vi "SingleDeviceDServer.vi"() -> ()   [LabVIEW 2014, in "examples.lvlib"]
uses:
  examples.lvlib
  vis/tango_vi.llb/_TangoState_t.ctl
  vis/tango_vi.llb/_DServerClientRequest.ctl
  vis/tango_vi.llb/_DServerClientRequestType.ctl
  vis/tango_vi.llb/_DServerClientRequestData.ctl
  vis/tango_vi.llb/_GenericDataBuffer.ctl
  vis/tango_vi.llb/_AttributeDataType_t.ctl
  vis/tango_vi.llb/_LoggingLevel.ctl
  vis/tango_vi.llb/_DServerDevicePropertyToDouble.vi
  vis/tango_vi.llb/_DServerRequestDataToDevBoolean.vi
  vis/tango_vi.llb/_DServerRequestDataFromDevBoolean.vi
  vis/tango_vi.llb/_DServerRequestDataToDevCharArray.vi
  vis/tango_vi.llb/_DServerRequestDataFromDevCharArray.vi
  vis/tango_vi.llb/_DServerRequestDataToDevDouble.vi
  vis/tango_vi.llb/_DServerRequestDataFromDevDouble.vi
  vis/tango_vi.llb/_DServerRequestDataToDevDoubleArray.vi
  vis/tango_vi.llb/_DServerRequestDataFromDevDoubleArray.vi
  vis/tango_vi.llb/_DServerRequestDataToDevDoubleStringArray.vi
  vis/tango_vi.llb/_DServerRequestDataFromDevDoubleStringArray.vi
  vis/tango_vi.llb/_DServerRequestDataToDevFloat.vi
  vis/tango_vi.llb/_DServerRequestDataFromDevFloat.vi
  vis/tango_vi.llb/_DServerRequestDataToDevFloatArray.vi
  vis/tango_vi.llb/_DServerRequestDataFromDevFloatArray.vi
  vis/tango_vi.llb/_DServerRequestDataToDevLong.vi
  vis/tango_vi.llb/_DServerRequestDataFromDevLong.vi
  vis/tango_vi.llb/_DServerRequestDataToDevLong64.vi
  vis/tango_vi.llb/_DServerRequestDataFromDevLong64.vi
  vis/tango_vi.llb/_DServerRequestDataToDevLong64Array.vi
  vis/tango_vi.llb/_DServerRequestDataFromDevLong64Array.vi
  vis/tango_vi.llb/_DServerRequestDataToDevLongArray.vi
  vis/tango_vi.llb/_DServerRequestDataFromDevLongArray.vi
  vis/tango_vi.llb/_DServerRequestDataToDevLongStringArray.vi
  vis/tango_vi.llb/_DServerRequestDataFromDevLongStringArray.vi
  vis/tango_vi.llb/_DServerRequestDataToDevShort.vi
  vis/tango_vi.llb/_DServerRequestDataFromDevShort.vi
  vis/tango_vi.llb/_DServerRequestDataToDevEnum.vi
  vis/tango_vi.llb/_DServerRequestDataFromDevEnum.vi
  vis/tango_vi.llb/_DServerRequestDataToDevShortArray.vi
  vis/tango_vi.llb/_DServerRequestDataFromDevShortArray.vi
  vis/tango_vi.llb/_DServerRequestDataToDevString.vi
  vis/tango_vi.llb/_DServerRequestDataFromDevString.vi
  vis/tango_vi.llb/_DServerRequestDataToDevStringArray.vi
  vis/tango_vi.llb/_DServerRequestDataFromDevStringArray.vi
  vis/tango_vi.llb/_DServerRequestDataToDevULong.vi
  vis/tango_vi.llb/_DServerRequestDataFromDevULong.vi
  vis/tango_vi.llb/_DServerRequestDataToDevULong64.vi
  vis/tango_vi.llb/_DServerRequestDataFromDevULong64.vi
  vis/tango_vi.llb/_DServerRequestDataToDevULong64Array.vi
  vis/tango_vi.llb/_DServerRequestDataFromDevULong64Array.vi
  vis/tango_vi.llb/_DServerRequestDataToDevULongArray.vi
  vis/tango_vi.llb/_DServerRequestDataFromDevULongArray.vi
  vis/tango_vi.llb/_DServerRequestDataToDevUShort.vi
  vis/tango_vi.llb/_DServerRequestDataFromDevUShort.vi
  AttributesDataStorage.vi
  Common/UtilsRandomInstances/_UtilsRandom2DBoolArray.vi
  vis/tango_vi.llb/_DServerSetBooleanImageAttributeValue.vi
  vis/tango_vi.llb/_DServerSetBooleanScalarAttributeValue.vi
  Common/UtilsRandomInstances/_UtilsRandomBoolArray.vi
  vis/tango_vi.llb/_DServerSetBooleanSpectrumAttributeValue.vi
  Common/UtilsRandomInstances/_UtilsRandom2DDBLArray.vi
  vis/tango_vi.llb/_DServerSetDoubleImageAttributeValue.vi
  vis/tango_vi.llb/_DServerSetDoubleScalarAttributeValue.vi
  Common/UtilsRandomInstances/_UtilsRandomDBLArray.vi
  vis/tango_vi.llb/_DServerSetDoubleSpectrumAttributeValue.vi
  Common/UtilsRandomInstances/_UtilsRandomI16Value.vi
  vis/tango_vi.llb/_DServerSetUShortScalarAttributeValue.vi
  Common/UtilsRandomInstances/_UtilsRandom2DSGLArray.vi
  vis/tango_vi.llb/_DServerSetFloatImageAttributeValue.vi
  Common/UtilsRandomInstances/_UtilsRandomSGLValue.vi
  vis/tango_vi.llb/_DServerSetFloatScalarAttributeValue.vi
  Common/UtilsRandomInstances/_UtilsRandomSGLArray.vi
  vis/tango_vi.llb/_DServerSetFloatSpectrumAttributeValue.vi
  Common/UtilsRandomInstances/_UtilsRandom2DI64Array.vi
  vis/tango_vi.llb/_DServerSetLong64ImageAttributeValue.vi
  Common/UtilsRandomInstances/_UtilsRandomI64Value.vi
  vis/tango_vi.llb/_DServerSetLong64ScalarAttributeValue.vi
  Common/UtilsRandomInstances/_UtilsRandomI64Array.vi
  vis/tango_vi.llb/_DServerSetLong64SpectrumAttributeValue.vi
  Common/UtilsRandomInstances/_UtilsRandom2DI32Array.vi
  vis/tango_vi.llb/_DServerSetLongImageAttributeValue.vi
  Common/UtilsRandomInstances/_UtilsRandomI32Value.vi
  vis/tango_vi.llb/_DServerSetLongScalarAttributeValue.vi
  Common/UtilsRandomInstances/_UtilsRandomU32Array.vi
  vis/tango_vi.llb/_DServerSetLongSpectrumAttributeValue.vi
  Common/UtilsRandomInstances/_UtilsRandom2DI16Array.vi
  vis/tango_vi.llb/_DServerSetShortImageAttributeValue.vi
  vis/tango_vi.llb/_DServerSetEnumScalarAttributeValue.vi
  Common/UtilsRandomInstances/_UtilsRandomI16Array.vi
  vis/tango_vi.llb/_DServerSetShortSpectrumAttributeValue.vi
  vis/tango_vi.llb/_DServerSetStateImageAttributeValue.vi
  vis/tango_vi.llb/_DServerSetStateScalarAttributeValue.vi
  vis/tango_vi.llb/_DServerSetStateSpectrumAttributeValue.vi
  vis/tango_vi.llb/_DServerSetStringImageAttributeValue.vi
  Common/UtilsRandomInstances/_UtilsRandomStringValue.vi
  vis/tango_vi.llb/_DServerSetStringScalarAttributeValue.vi
  vis/tango_vi.llb/_DServerSetStringSpectrumAttributeValue.vi
  Common/UtilsRandomInstances/_UtilsRandom2DU8Array.vi
  vis/tango_vi.llb/_DServerSetUCharImageAttributeValue.vi
  Common/UtilsRandomInstances/_UtilsRandomU8Value.vi
  vis/tango_vi.llb/_DServerSetUCharScalarAttributeValue.vi
  Common/UtilsRandomInstances/_UtilsRandomU8Array.vi
  vis/tango_vi.llb/_DServerSetUCharSpectrumAttributeValue.vi
  Common/UtilsRandomInstances/_UtilsRandom2DU64Array.vi
  vis/tango_vi.llb/_DServerSetULong64ImageAttributeValue.vi
  Common/UtilsRandomInstances/_UtilsRandomU64Value.vi
  vis/tango_vi.llb/_DServerSetULong64ScalarAttributeValue.vi
  Common/UtilsRandomInstances/_UtilsRandomU64Array.vi
  vis/tango_vi.llb/_DServerSetULong64SpectrumAttributeValue.vi
  Common/UtilsRandomInstances/_UtilsRandom2DU32Array.vi
  vis/tango_vi.llb/_DServerSetULongImageAttributeValue.vi
  Common/UtilsRandomInstances/_UtilsRandomU32Value.vi
  vis/tango_vi.llb/_DServerSetULongScalarAttributeValue.vi
  Common/UtilsRandomInstances/_UtilsRandomI32Array.vi
  vis/tango_vi.llb/_DServerSetULongSpectrumAttributeValue.vi
  Common/UtilsRandomInstances/_UtilsRandom2DU16Array.vi
  vis/tango_vi.llb/_DServerSetUShortImageAttributeValue.vi
  Common/UtilsRandomInstances/_UtilsRandomU16Value.vi
  Common/UtilsRandomInstances/_UtilsRandomU16Array.vi
  vis/tango_vi.llb/_DServerSetUShortSpectrumAttributeValue.vi
  vis/tango_vi.llb/_DServerRequestDataToBooleanImage.vi
  vis/tango_vi.llb/_DServerRequestDataToBooleanScalar.vi
  vis/tango_vi.llb/_DServerRequestDataToBooleanSpectrum.vi
  vis/tango_vi.llb/_DServerRequestDataToDoubleImage.vi
  vis/tango_vi.llb/_DServerRequestDataToDoubleScalar.vi
  vis/tango_vi.llb/_DServerRequestDataToDoubleSpectrum.vi
  vis/tango_vi.llb/_DServerRequestDataToFloatImage.vi
  vis/tango_vi.llb/_DServerRequestDataToFloatScalar.vi
  vis/tango_vi.llb/_DServerRequestDataToFloatSpectrum.vi
  vis/tango_vi.llb/_DServerRequestDataToLong64Image.vi
  vis/tango_vi.llb/_DServerRequestDataToLong64Scalar.vi
  vis/tango_vi.llb/_DServerRequestDataToLong64Spectrum.vi
  vis/tango_vi.llb/_DServerRequestDataToLongImage.vi
  vis/tango_vi.llb/_DServerRequestDataToLongScalar.vi
  vis/tango_vi.llb/_DServerRequestDataToLongSpectrum.vi
  vis/tango_vi.llb/_DServerRequestDataToShortImage.vi
  vis/tango_vi.llb/_DServerRequestDataToShortScalar.vi
  vis/tango_vi.llb/_DServerRequestDataToEnumScalar.vi
  vis/tango_vi.llb/_DServerRequestDataToShortSpectrum.vi
  vis/tango_vi.llb/_DServerRequestDataToStateImage.vi
  vis/tango_vi.llb/_DServerRequestDataToStateScalar.vi
  vis/tango_vi.llb/_DServerRequestDataToStateSpectrum.vi
  vis/tango_vi.llb/_DServerRequestDataToStringImage.vi
  vis/tango_vi.llb/_DServerRequestDataToStringScalar.vi
  vis/tango_vi.llb/_DServerRequestDataToStringSpectrum.vi
  vis/tango_vi.llb/_DServerRequestDataToUCharImage.vi
  vis/tango_vi.llb/_DServerRequestDataToUCharScalar.vi
  vis/tango_vi.llb/_DServerRequestDataToUCharSpectrum.vi
  vis/tango_vi.llb/_DServerRequestDataToULong64Spectrum.vi
  vis/tango_vi.llb/_DServerRequestDataToULong64Scalar.vi
  vis/tango_vi.llb/_DServerRequestDataToULongImage.vi
  vis/tango_vi.llb/_DServerRequestDataToULongScalar.vi
  vis/tango_vi.llb/_DServerRequestDataToULongSpectrum.vi
  vis/tango_vi.llb/_DServerRequestDataToUShortImage.vi
  vis/tango_vi.llb/_DServerRequestDataToUShortScalar.vi
  vis/tango_vi.llb/_DServerRequestDataToUShortSpectrum.vi
  vis/tango_vi.llb/tango.lvlib
panel:
  in  "Device Tmo (in sec)":dbl=3.0
  out "Scale [Property Val.]":dbl
  out "Client Request":T1={"Request Id"=0, "Source Id"=0, "Request Type"=enum."UNKNOWN_REQUEST", "Device Class Name"="unspecified_class_name", "Device Name"="unspecified/device/name", "Cmd or Attr Name"="unspecified_cmd_or_attr_name", "Client Request Data"={"write attribute value"={"dimx"=0, "dimy"=0, "data"=[], "data_type"=enum."UNKNOWN_DATA_TYPE"}, "exec. command argin"={"num data"=[], "str data"=[]}}}
  out "State":T6=enum."UNKNOWN"
  out "Devive List":string[](array[string])
  in  "Instance Name":string="1"
  in  "Executable Name":string="LabviewSingleDeviceDServer"
  in  "devDoubleScalar":dbl(knob)=50.0 max=400.0 scale=0.0..100.0
  in  "?":bool
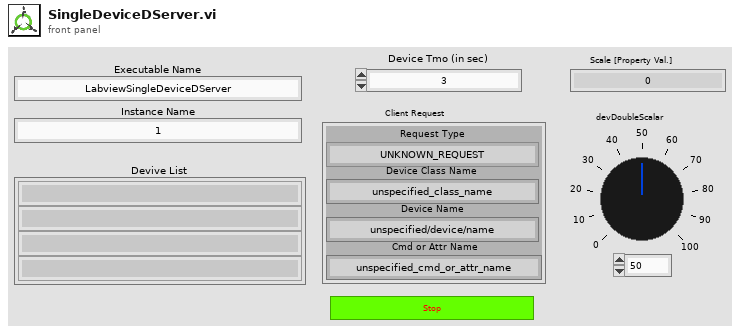
[diagram p1: front panel]
types:
  T1 = typedef "tango.lvlib/_DServerClientRequest.ctl" = cluster{"Request Id":u32, "Source Id":u32, "Request Type":T2, "Device Class Name":string, "Device Name":string, "Cmd or Attr Name":string, "Client Request Data":T3}
  T2 = typedef "tango.lvlib/_DServerClientRequestType.ctl" = enum16{"EXEC_CMD", "READ_ATTR", "WRITE_ATTR", "UNKNOWN_REQUEST"}
  T3 = typedef "tango.lvlib/_DServerClientRequestData.ctl" = cluster{"write attribute value":T4, "exec. command argin":cluster{"num data":u8[], "str data":string[]}}
  T4 = typedef "tango.lvlib/_GenericDataBuffer.ctl" = cluster{"dimx":u32, "dimy":u32, "data":u8[], "data_type":T5}
  T5 = typedef "tango.lvlib/_AttributeDataType_t.ctl" = enum16{"STATE_SCA", "STATE_SPE", "STATE_IMG", "STRING_SCA", "STRING_SPE", "STRING_IMG", "BOOL_SCA", "BOOL_SPE", "BOOL_IMG", "UCHAR_SCA", "UCHAR_SPE", "UCHAR_IMG", "SHORT_SCA", "SHORT_SPE", "SHORT_IMG", "USHORT_SCA", "USHORT_SPE", "USHORT_IMG", "LONG_SCA", "LONG_SPE", "LONG_IMG", "ULONG_SCA", "ULONG_SPE", "ULONG_IMG", "LONG64_SCA", "LONG64_SPE", "LONG64_IMG", "ULONG64_SCA", "ULONG64_SPE", "ULONG64_IMG", "FLOAT_SCA", "FLOAT_SPE", "FLOAT_IMG", "DOUBLE_SCA", "DOUBLE_SPE", "DOUBLE_IMG", "ENUM_SCA", "UNKNOWN_DATA_TYPE"}
  T6 = typedef "tango.lvlib/_TangoState_t.ctl" = enum32{"ON", "OFF", "CLOSE", "OPEN", "INSERT", "EXTRACT", "MOVING", "STANDBY", "FAULT", "INIT", "RUNNING", "ALARM", "DISABLE", "UNKNOWN"}
  T7 = typedef "tango.lvlib/_DServerEvent.ctl" = cluster{"event registration refnum":refnum<event-registration>, "user event out":refnum<user-event>}
  T8 = typedef "tango.lvlib/_LoggingLevel.ctl" = enum16{"DEBUG", "INFO", "WARNING", "ERROR", "FATAL"}
  T9 = enum16{"ENUM0", "ENUM1", "ENUM2", "ENUM3", "UNKNOWN"}
  T10 = cluster{"device name":string, "attribute name":string, "r/w access":i16, "format":i16, "data type":i16, "level":i16, "label":string, "unit":string, "display format":string, "min value":string, "max value":string, "min alarm":string, "max alarm":string}
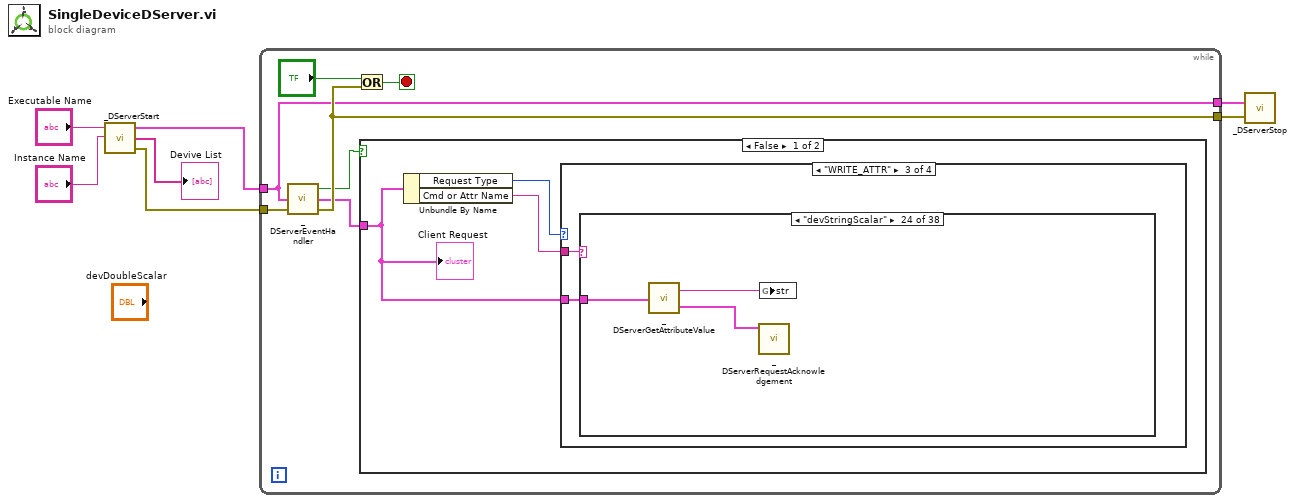
[diagram p0: block diagram]
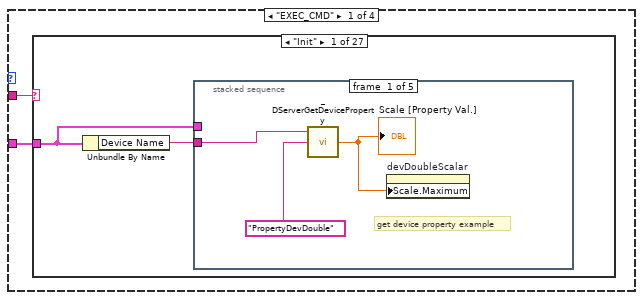
[diagram p2: hidden frame]
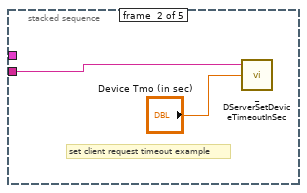
[diagram p3: hidden frame]
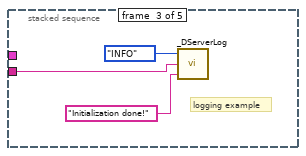
[diagram p4: hidden frame]
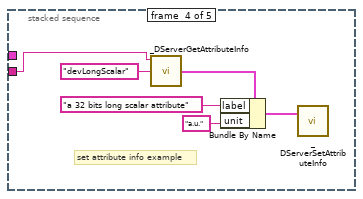
[diagram p5: hidden frame]
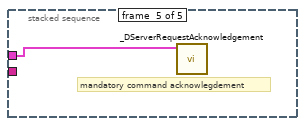
[diagram p6: hidden frame]
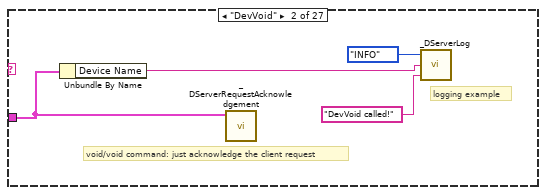
[diagram p7: hidden frame]
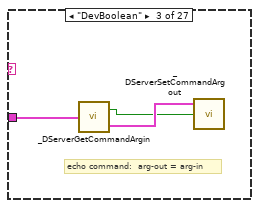
[diagram p8: hidden frame]
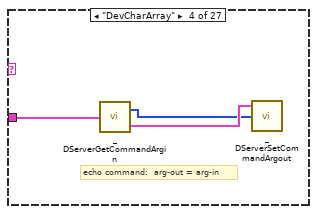
[diagram p9: hidden frame]
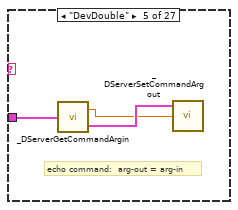
[diagram p10: hidden frame]
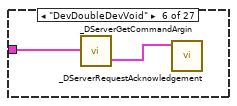
[diagram p11: hidden frame]
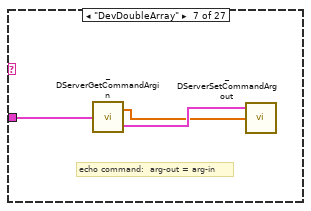
[diagram p12: hidden frame]
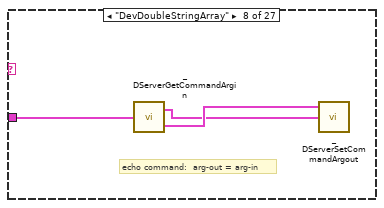
[diagram p13: hidden frame]
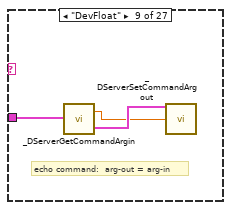
[diagram p14: hidden frame]
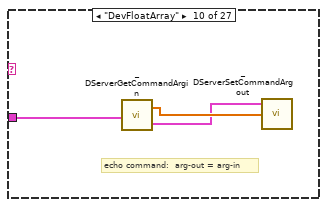
[diagram p15: hidden frame]
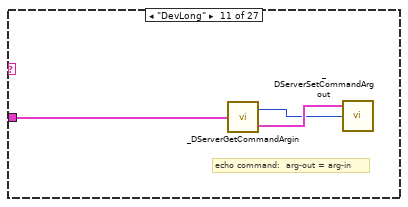
[diagram p16: hidden frame]
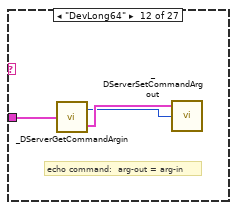
[diagram p17: hidden frame]
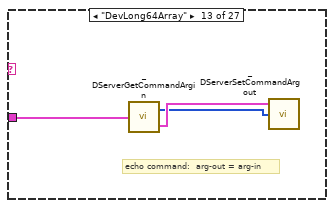
[diagram p18: hidden frame]
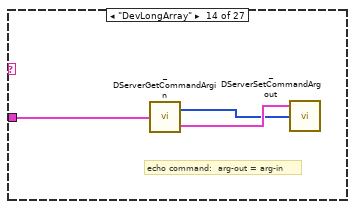
[diagram p19: hidden frame]
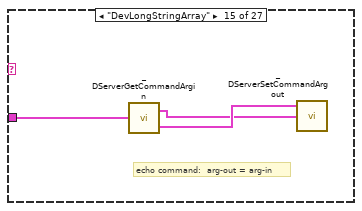
[diagram p20: hidden frame]
diagram:
  n1 = call "_DServerStart.vi"("instance name"="Instance Name", "executable name"="Executable Name") -> ("error out"=w5:errorcluster, "device_list"=→"Devive List":string[], "dserver evt."=w7:T7)  [unwired: 1 in]
  n2 = while {
    tunnel: w5 -> [w12]
    tunnel: w7 -> [w10]
    tunnel: [w11] -> w2
    tunnel: [w10] -> w1
    stop <- w14 stop-if-true
    n3 = call "_DServerEventHandler.vi"("error in"=w12, "dserver evt."=w10) -> ("error out"=w11:errorcluster, "client request"=w8:T1, "timeout"=w9:bool)  [unwired: 1 in]
    n4 = Or(x="?", y=w11) -> (x .or. y?=w14:bool)
    n5 = case shown="False" w9 {
      tunnel: w8 -> [w15 _]
      frame False {
        n6 = Unbundle By Name(w15) -> ("Request Type"=w16:T2, "Cmd or Attr Name"=w17:string)
        n7 = case shown="\"WRITE_ATTR\"" w16 {
          tunnel: w17 -> [w19 w114 w400 _]
          tunnel: w15 -> [w18 w113 w399 w513]
          frame "EXEC_CMD" {
            n8 = case shown="\"Init\"" w19 {
              tunnel: w18 -> [w20 w37 w41 w46 w49 w51 w54 w57 w60 w63 w64 w67 w71 w75 w76 w81 w84 w87 w90 w93 w96 w97 w102 w105 w108 w111 w112]
              frame "Init" {
                n9 = Unbundle By Name(w20) -> ("Device Name"=w21:string)
                n10 = stacked-sequence {
                  tunnel: w21 -> [w23 w25 w28 w32 _]
                  tunnel: w20 -> [_ _ _ _ w36]
                  frame #0 {
                    # "get device property example"
                    n11 = call-poly "_DServerGetDeviceProperty.vi"("property name"="PropertyDevDouble", "device name"=w23) -> ("property value"=w22:dbl)  [unwired: 2 in, 1 out]
                    "Scale [Property Val.]" <- w22
                    n12 = property on="devDoubleScalar" class="Knob (strict)"("Scale.Maximum"=w22) -> ()  [unwired: 2 in, 2 out]
                  }
                  frame #1 {
                    # "set client request timeout example"
                    n13 = call "_DServerSetDeviceTimeoutInSec.vi"("client request timeout in sec"="Device Tmo (in sec)", "device name"=w25) -> ()  [unwired: 3 in, 1 out]
                  }
                  frame #2 {
                    # "logging example"
                    n14 = call "_DServerLog.vi"("text"="Initialization done!", "device name"=w28, "logging level"=_LoggingLevel."INFO") -> ()  [unwired: 3 in]
                  }
                  frame #3 {
                    # "set attribute info example"
                    n15 = call "_DServerGetAttributeInfo.vi"("attribute name"="devLongScalar", "device name"=w32) -> ("attribute info"=w34:T10)  [unwired: 2 in, 1 out]
                    n16 = Bundle By Name(cluster=w34, "label"="a 32 bits long scalar attribute", "unit"="a.u.") -> (w33:T10)
                    n17 = call "_DServerSetAttributeInfo.vi"("attribute info"=w33) -> ()  [unwired: 2 in, 1 out]
                  }
                  frame #4 {
                    # "mandatory command acknowlegdement"
                    n18 = call "_DServerRequestAcknowledgement.vi"("client request"=w36) -> ()  [unwired: 6 in, 1 out]
                  }
                }
              }
              frame "DevVoid" {
                # "logging example"
                # "void/void command: just acknowledge the client request"
                n19 = Unbundle By Name(w37) -> ("Device Name"=w38:string)
                n20 = call "_DServerRequestAcknowledgement.vi"("client request"=w37) -> ()  [unwired: 6 in, 1 out]
                n21 = call "_DServerLog.vi"("text"="DevVoid called!", "device name"=w38, "logging level"=_LoggingLevel."INFO") -> ()  [unwired: 3 in]
              }
              frame "DevBoolean" {
                # "echo command:  arg-out = arg-in"
                n22 = call-poly "_DServerGetCommandArgin.vi"("client request"=w41) -> ("argin"=w42:bool, "client request"=w43:T1)
                n23 = call-poly "_DServerSetCommandArgout.vi"("argout value"=w42, "client request"=w43) -> ()  [unwired: 3 in, 1 out]
              }
              frame "DevCharArray" {
                # "echo command:  arg-out = arg-in"
                n24 = call-poly "_DServerGetCommandArgin.vi"("client request"=w46) -> ("argin"=w44:i8[], "client request"=w45:T1)
                n25 = call-poly "_DServerSetCommandArgout.vi"("argout value"=w44, "client request"=w45) -> ()  [unwired: 3 in, 1 out]
              }
              frame "DevDouble" {
                # "echo command:  arg-out = arg-in"
                n26 = call-poly "_DServerGetCommandArgin.vi"("client request"=w49) -> ("argin"=w47:dbl, "client request"=w48:T1)
                n27 = call-poly "_DServerSetCommandArgout.vi"("argout value"=w47, "client request"=w48) -> ()  [unwired: 3 in, 1 out]
              }
              frame "DevDoubleDevVoid" {
                n28 = call-poly "_DServerGetCommandArgin.vi"("client request"=w51) -> ("client request"=w50:T1)  [unwired: 1 out]
                n29 = call "_DServerRequestAcknowledgement.vi"("client request"=w50) -> ()  [unwired: 6 in, 1 out]
              }
              frame "DevDoubleArray" {
                # "echo command:  arg-out = arg-in"
                n30 = call-poly "_DServerGetCommandArgin.vi"("client request"=w54) -> ("argin"=w52:dbl[], "client request"=w53:T1)
                n31 = call-poly "_DServerSetCommandArgout.vi"("argout value"=w52, "client request"=w53) -> ()  [unwired: 3 in, 1 out]
              }
              frame "DevDoubleStringArray" {
                # "echo command:  arg-out = arg-in"
                n32 = call-poly "_DServerGetCommandArgin.vi"("client request"=w57) -> ("argin"=w55:cluster{"dvalue":dbl[], "svalue":string[]}, "client request"=w56:T1)
                n33 = call-poly "_DServerSetCommandArgout.vi"("argout value"=w55, "client request"=w56) -> ()  [unwired: 3 in, 1 out]
              }
              frame "DevFloat" {
                # "echo command:  arg-out = arg-in"
                n34 = call-poly "_DServerGetCommandArgin.vi"("client request"=w60) -> ("argin"=w58:sgl, "client request"=w59:T1)
                n35 = call-poly "_DServerSetCommandArgout.vi"("argout value"=w58, "client request"=w59) -> ()  [unwired: 3 in, 1 out]
              }
              frame "DevFloatArray" {
                # "echo command:  arg-out = arg-in"
                n36 = call-poly "_DServerGetCommandArgin.vi"("client request"=w63) -> ("argin"=w62:sgl[], "client request"=w61:T1)
                n37 = call-poly "_DServerSetCommandArgout.vi"("argout value"=w62, "client request"=w61) -> ()  [unwired: 3 in, 1 out]
              }
              frame "DevLong" {
                # "echo command:  arg-out = arg-in"
                n38 = call-poly "_DServerGetCommandArgin.vi"("client request"=w64) -> ("argin"=w65:i32, "client request"=w66:T1)
                n39 = call-poly "_DServerSetCommandArgout.vi"("argout value"=w65, "client request"=w66) -> ()  [unwired: 3 in, 1 out]
              }
              frame "DevLong64" {
                # "echo command:  arg-out = arg-in"
                n40 = call-poly "_DServerGetCommandArgin.vi"("client request"=w67) -> ("argin"=w68:i64, "client request"=w69:T1)
                n41 = call-poly "_DServerSetCommandArgout.vi"("argout value"=w68, "client request"=w69) -> ()  [unwired: 3 in, 1 out]
              }
              frame "DevLong64Array" {
                # "echo command:  arg-out = arg-in"
                n42 = call-poly "_DServerGetCommandArgin.vi"("client request"=w71) -> ("argin"=w70:i64[], "client request"=w72:T1)
                n43 = call-poly "_DServerSetCommandArgout.vi"("argout value"=w70, "client request"=w72) -> ()  [unwired: 3 in, 1 out]
              }
              frame "DevLongArray" {
                # "echo command:  arg-out = arg-in"
                n44 = call-poly "_DServerGetCommandArgin.vi"("client request"=w75) -> ("argin"=w73:i32[], "client request"=w74:T1)
                n45 = call-poly "_DServerSetCommandArgout.vi"("argout value"=w73, "client request"=w74) -> ()  [unwired: 3 in, 1 out]
              }
              frame "DevLongStringArray" {
                # "echo command:  arg-out = arg-in"
                n46 = call-poly "_DServerGetCommandArgin.vi"("client request"=w76) -> ("argin"=w77:cluster{"lvalue":i32[], "svalue":string[]}, "client request"=w78:T1)
                n47 = call-poly "_DServerSetCommandArgout.vi"("argout value"=w77, "client request"=w78) -> ()  [unwired: 3 in, 1 out]
              }
              frame "DevShort" {
                # "echo command:  arg-out = arg-in"
                n48 = call-poly "_DServerGetCommandArgin.vi"("client request"=w81) -> ("argin"=w79:i16, "client request"=w80:T1)
                n49 = call-poly "_DServerSetCommandArgout.vi"("argout value"=w79, "client request"=w80) -> ()  [unwired: 3 in, 1 out]
              }
              frame "DevEnum" {
                # "echo command:  arg-out = arg-in"
                n50 = call-poly "_DServerGetCommandArgin.vi"("client request"=w84) -> ("argin"=w82:i16, "client request"=w83:T1)
                n51 = call-poly "_DServerSetCommandArgout.vi"("argout value"=w82, "client request"=w83) -> ()  [unwired: 3 in, 1 out]
              }
              frame "DevShortArray" {
                # "echo command:  arg-out = arg-in"
                n52 = call-poly "_DServerGetCommandArgin.vi"("client request"=w87) -> ("argin"=w85:i16[], "client request"=w86:T1)
                n53 = call-poly "_DServerSetCommandArgout.vi"("argout value"=w85, "client request"=w86) -> ()  [unwired: 3 in, 1 out]
              }
              frame "DevString" {
                # "echo command:  arg-out = arg-in"
                n54 = call-poly "_DServerGetCommandArgin.vi"("client request"=w90) -> ("argin"=w88:string, "client request"=w89:T1)
                n55 = call-poly "_DServerSetCommandArgout.vi"("argout value"=w88, "client request"=w89) -> ()  [unwired: 3 in, 1 out]
              }
              frame "DevStringArray" {
                # "echo command:  arg-out = arg-in"
                n56 = call-poly "_DServerGetCommandArgin.vi"("client request"=w93) -> ("argin"=w91:string[], "client request"=w92:T1)
                n57 = call-poly "_DServerSetCommandArgout.vi"("argout value"=w91, "client request"=w92) -> ()  [unwired: 3 in, 1 out]
              }
              frame "DevULong" {
                # "echo command:  arg-out = arg-in"
                n58 = call-poly "_DServerGetCommandArgin.vi"("client request"=w96) -> ("argin"=w94:u32, "client request"=w95:T1)
                n59 = call-poly "_DServerSetCommandArgout.vi"("argout value"=w94, "client request"=w95) -> ()  [unwired: 3 in, 1 out]
              }
              frame "DevULong64" {
                # "echo command:  arg-out = arg-in"
                n60 = call-poly "_DServerGetCommandArgin.vi"("client request"=w97) -> ("argin"=w98:u64, "client request"=w99:T1)
                n61 = call-poly "_DServerSetCommandArgout.vi"("argout value"=w98, "client request"=w99) -> ()  [unwired: 3 in, 1 out]
              }
              frame "DevULong64Array" {
                # "echo command:  arg-out = arg-in"
                n62 = call-poly "_DServerGetCommandArgin.vi"("client request"=w102) -> ("argin"=w100:u64[], "client request"=w101:T1)
                n63 = call-poly "_DServerSetCommandArgout.vi"("argout value"=w100, "client request"=w101) -> ()  [unwired: 3 in, 1 out]
              }
              frame "DevULongArray" {
                # "echo command:  arg-out = arg-in"
                n64 = call-poly "_DServerGetCommandArgin.vi"("client request"=w105) -> ("argin"=w103:u32[], "client request"=w104:T1)
                n65 = call-poly "_DServerSetCommandArgout.vi"("argout value"=w103, "client request"=w104) -> ()  [unwired: 3 in, 1 out]
              }
              frame "DevUShort" {
                # "echo command:  arg-out = arg-in"
                n66 = call-poly "_DServerGetCommandArgin.vi"("client request"=w108) -> ("argin"=w106:u16, "client request"=w107:T1)
                n67 = call-poly "_DServerSetCommandArgout.vi"("argout value"=w106, "client request"=w107) -> ()  [unwired: 3 in, 1 out]
              }
              frame "DevUShortArray" {
                # "echo command:  arg-out = arg-in"
                n68 = call-poly "_DServerGetCommandArgin.vi"("client request"=w111) -> ("argin"=w109:i16[], "client request"=w110:T1)
                n69 = call-poly "_DServerSetCommandArgout.vi"("argout value"=w109, "client request"=w110) -> ()  [unwired: 3 in, 1 out]
              }
              frame Default {
                # "oops, this client request is not implemented"
                n70 = call "_DServerUnimplementedRequest.vi"("client request"=w112) -> ()  [unwired: 2 in, 1 out]
              }
            }
          }
          frame "READ_ATTR" {
            n71 = case shown="\"devBooleanImage\"" w114 {
              tunnel: w113 -> [w115 w124 w126 w133 w142 w144 w151 w160 w169 w175 w182 w191 w197 w204 w213 w219 w227 w235 w242 w248 w253 w255 w259 w271 w278 w288 w297 w304 w310 w319 w325 w332 w341 w347 w354 w363 w369 _ w376 w384 w392 w397 w398]
              frame "devBooleanImage" {
                # "return last written value or a random one in \n  case the attribute has never been written"
                n72 = global read "AttributesDataStorage.vi" "booli"() -> (w121:bool[][])
                n73 = Array Size(array=w121) -> (size(s)=w118:i32[])
                n74 = Index Array(array=w118, index=0) -> (element=w120:i32)
                n75 = Not Equal To 0?(x=w120) -> (x != 0?=w117:bool)
                n76 = case shown="False" w117 {
                  tunnel: [w122 w123] -> w116
                  tunnel: w121 -> [_ w123]
                  frame False {
                    n77 = call-poly "Random2DArray.vi"() -> ("random array"=w122:bool[][])  [unwired: 2 in]
                  }
                  frame True {
                  }
                }
                n78 = call-poly "_DServerSetAttributeValue.vi"("value"=w116, "client request"=w115) -> ()  [unwired: 3 in, 1 out]
              }
              frame "devBooleanScalar" {
                n79 = global read "AttributesDataStorage.vi" "bool"() -> (w125:bool)
                n80 = call-poly "_DServerSetAttributeValue.vi"(4:w125, "client request"=w124) -> ()  [unwired: 3 in, 1 out]
              }
              frame "devBooleanSpectrum" {
                # "return last written value or a random one in \n  case the attribute has never been written"
                n81 = global read "AttributesDataStorage.vi" "boolsp"() -> (w128:bool[])
                n82 = Array Size(array=w128) -> (size(s)=w129:i32)
                n83 = Not Equal To 0?(x=w129) -> (x != 0?=w130:bool)
                n84 = case shown="False" w130 {
                  tunnel: [w131 w132] -> w127
                  tunnel: w128 -> [_ w132]
                  frame False {
                    n85 = call-poly "Random1DArray.vi"() -> ("array"=w131:bool[])  [unwired: 2 in]
                  }
                  frame True {
                  }
                }
                n86 = call-poly "_DServerSetAttributeValue.vi"("value"=w127, "client request"=w126) -> ()  [unwired: 3 in, 1 out]
              }
              frame "devDoubleImage" {
                # "return last written value or a random one in \n  case the attribute has never been written"
                n87 = global read "AttributesDataStorage.vi" "dbli"() -> (w139:dbl[][])
                n88 = Array Size(array=w139) -> (size(s)=w136:i32[])
                n89 = Index Array(array=w136, index=0) -> (element=w138:i32)
                n90 = Not Equal To 0?(x=w138) -> (x != 0?=w135:bool)
                n91 = case shown="False" w135 {
                  tunnel: [w140 w141] -> w134
                  tunnel: w139 -> [_ w141]
                  frame False {
                    n92 = call-poly "Random2DArray.vi"() -> ("random array"=w140:dbl[][])  [unwired: 2 in]
                  }
                  frame True {
                  }
                }
                n93 = call-poly "_DServerSetAttributeValue.vi"("value"=w134, "client request"=w133) -> ()  [unwired: 3 in, 1 out]
              }
              frame "devDoubleScalar" {
                n94 = property on="devDoubleScalar" class="Knob (strict)"() -> ("Value"=w143:dbl)  [unwired: 2 in, 2 out]
                n95 = call-poly "_DServerSetAttributeValue.vi"("value"=w143, "client request"=w142) -> ()  [unwired: 3 in, 1 out]
              }
              frame "devDoubleSpectrum" {
                # "return last written value or a random one in \n  case the attribute has never been written"
                n96 = global read "AttributesDataStorage.vi" "dblsp"() -> (w146:dbl[])
                n97 = Array Size(array=w146) -> (size(s)=w147:i32)
                n98 = Not Equal To 0?(x=w147) -> (x != 0?=w148:bool)
                n99 = case shown="True" w148 {
                  tunnel: [w149 w150] -> w145
                  tunnel: w146 -> [_ w150]
                  frame False {
                    n100 = call-poly "Random1DArray.vi"() -> ("array"=w149:dbl[])  [unwired: 2 in]
                  }
                  frame True {
                  }
                }
                n101 = call-poly "_DServerSetAttributeValue.vi"("value"=w145, "client request"=w144) -> ()  [unwired: 3 in, 1 out]
              }
              frame "devEnumScalar" {
                # "return last written value or a random one in \n  case the attribute has never been written"
                n102 = global read "AttributesDataStorage.vi" "enum"() -> (w154:T9)
                n103 = Not Equal?(x=T9."UNKNOWN", y=w154) -> (x != y?=w155:bool)
                n104 = case shown="False" w155 {
                  tunnel: [w157 w159] -> w152
                  tunnel: w154 -> [_ w159]
                  frame False {
                    n105 = call-poly "RandomScalar.vi"() -> ("random value"=w158:i16)  [unwired: 1 in]
                    n106 = Quotient & Remainder(x=w158, y=T9."UNKNOWN" ("x")) -> (x-y*floor(x/y)=w157:u16)  [unwired: 1 out]
                  }
                  frame True {
                  }
                }
                n107 = call-poly "_DServerSetAttributeValue.vi"("value"=w152, "client request"=w151) -> ()  [unwired: 3 in, 1 out]
              }
              frame "devFloatImage" {
                # "return last written value or a random one in \n  case the attribute has never been written"
                n108 = global read "AttributesDataStorage.vi" "sgli"() -> (w166:sgl[][])
                n109 = Array Size(array=w166) -> (size(s)=w163:i32[])
                n110 = Index Array(array=w163, index=0) -> (element=w165:i32)
                n111 = Not Equal To 0?(x=w165) -> (x != 0?=w162:bool)
                n112 = case shown="False" w162 {
                  tunnel: [w167 w168] -> w161
                  tunnel: w166 -> [_ w168]
                  frame False {
                    n113 = call-poly "Random2DArray.vi"() -> ("random array"=w167:sgl[][])  [unwired: 2 in]
                  }
                  frame True {
                  }
                }
                n114 = call-poly "_DServerSetAttributeValue.vi"("value"=w161, "client request"=w160) -> ()  [unwired: 3 in, 1 out]
              }
              frame "devFloatScalar" {
                # "return last written value or a random one in \n  case the attribute has never been written"
                n115 = global read "AttributesDataStorage.vi" "sgl"() -> (w171:sgl)
                n116 = Not Equal To 0?(x=w171) -> (x != 0?=w172:bool)
                n117 = case shown="False" w172 {
                  tunnel: [w173 w174] -> w170
                  tunnel: w171 -> [_ w174]
                  frame False {
                    n118 = call-poly "RandomScalar.vi"() -> ("random value"=w173:sgl)  [unwired: 1 in]
                  }
                  frame True {
                  }
                }
                n119 = call-poly "_DServerSetAttributeValue.vi"("value"=w170, "client request"=w169) -> ()  [unwired: 3 in, 1 out]
              }
              frame "devFloatSpectrum" {
                # "return last written value or a random one in \n  case the attribute has never been written"
                n120 = global read "AttributesDataStorage.vi" "sglsp"() -> (w177:sgl[])
                n121 = Array Size(array=w177) -> (size(s)=w178:i32)
                n122 = Not Equal To 0?(x=w178) -> (x != 0?=w179:bool)
                n123 = case shown="False" w179 {
                  tunnel: [w180 w181] -> w176
                  tunnel: w177 -> [_ w181]
                  frame False {
                    n124 = call-poly "Random1DArray.vi"() -> ("array"=w180:sgl[])  [unwired: 2 in]
                  }
                  frame True {
                  }
                }
                n125 = call-poly "_DServerSetAttributeValue.vi"("value"=w176, "client request"=w175) -> ()  [unwired: 3 in, 1 out]
              }
              frame "devLong64Image" {
                # "return last written value or a random one in \n  case the attribute has never been written"
                n126 = global read "AttributesDataStorage.vi" "i64i"() -> (w188:i64[][])
                n127 = Array Size(array=w188) -> (size(s)=w185:i32[])
                n128 = Index Array(array=w185, index=0) -> (element=w187:i32)
                n129 = Not Equal To 0?(x=w187) -> (x != 0?=w184:bool)
                n130 = case shown="False" w184 {
                  tunnel: [w189 w190] -> w183
                  tunnel: w188 -> [_ w190]
                  frame False {
                    n131 = call-poly "Random2DArray.vi"() -> ("random array"=w189:i64[][])  [unwired: 2 in]
                  }
                  frame True {
                  }
                }
                n132 = call-poly "_DServerSetAttributeValue.vi"("value"=w183, "client request"=w182) -> ()  [unwired: 3 in, 1 out]
              }
              frame "devLong64Scalar" {
                # "return last written value or a random one in \n  case the attribute has never been written"
                n133 = global read "AttributesDataStorage.vi" "i64"() -> (w193:i64)
                n134 = Not Equal To 0?(x=w193) -> (x != 0?=w194:bool)
                n135 = case shown="False" w194 {
                  tunnel: [w195 w196] -> w192
                  tunnel: w193 -> [_ w196]
                  frame False {
                    n136 = call-poly "RandomScalar.vi"() -> ("random value"=w195:i64)  [unwired: 1 in]
                  }
                  frame True {
                  }
                }
                n137 = call-poly "_DServerSetAttributeValue.vi"("value"=w192, "client request"=w191) -> ()  [unwired: 3 in, 1 out]
              }
              frame "devLong64Spectrum" {
                # "return last written value or a random one in \n  case the attribute has never been written"
                n138 = global read "AttributesDataStorage.vi" "i64sp"() -> (w199:i64[])
                n139 = Array Size(array=w199) -> (size(s)=w200:i32)
                n140 = Not Equal To 0?(x=w200) -> (x != 0?=w201:bool)
                n141 = case shown="False" w201 {
                  tunnel: [w202 w203] -> w198
                  tunnel: w199 -> [_ w203]
                  frame False {
                    n142 = call-poly "Random1DArray.vi"() -> ("array"=w202:i64[])  [unwired: 2 in]
                  }
                  frame True {
                  }
                }
                n143 = call-poly "_DServerSetAttributeValue.vi"("value"=w198, "client request"=w197) -> ()  [unwired: 3 in, 1 out]
              }
              frame "devLongImage" {
                # "return last written value or a random one in \n  case the attribute has never been written"
                n144 = global read "AttributesDataStorage.vi" "i32i"() -> (w210:i32[][])
                n145 = Array Size(array=w210) -> (size(s)=w207:i32[])
                n146 = Index Array(array=w207, index=0) -> (element=w209:i32)
                n147 = Not Equal To 0?(x=w209) -> (x != 0?=w206:bool)
                n148 = case shown="False" w206 {
                  tunnel: [w211 w212] -> w205
                  tunnel: w210 -> [_ w212]
                  frame False {
                    n149 = call-poly "Random2DArray.vi"() -> ("random array"=w211:i32[][])  [unwired: 2 in]
                  }
                  frame True {
                  }
                }
                n150 = call-poly "_DServerSetAttributeValue.vi"("value"=w205, "client request"=w204) -> ()  [unwired: 3 in, 1 out]
              }
              frame "devLongScalar" {
                # "return last written value or a random one in \n  case the attribute has never been written"
                n151 = global read "AttributesDataStorage.vi" "i32"() -> (w214:i32)
                n152 = Not Equal To 0?(x=w214) -> (x != 0?=w216:bool)
                n153 = case shown="False" w216 {
                  tunnel: [w217 w218] -> w215
                  tunnel: w214 -> [_ w218]
                  frame False {
                    n154 = call-poly "RandomScalar.vi"() -> ("random value"=w217:i32)  [unwired: 1 in]
                  }
                  frame True {
                  }
                }
                n155 = call-poly "_DServerSetAttributeValue.vi"("value"=w215, "client request"=w213) -> ()  [unwired: 3 in, 1 out]
              }
              frame "devLongSpectrum" {
                # "return last written value or a random one in \n  case the attribute has never been written"
                n156 = global read "AttributesDataStorage.vi" "i32sp"() -> (w221:i32[])
                n157 = Array Size(array=w221) -> (size(s)=w222:i32)
                n158 = Not Equal To 0?(x=w222) -> (x != 0?=w223:bool)
                n159 = case shown="False" w223 {
                  tunnel: [w224 w225] -> w220
                  tunnel: w221 -> [_ w225]
                  frame False {
                    n160 = call-poly "Random1DArray.vi"() -> ("array"=w224:i32[])  [unwired: 2 in]
                  }
                  frame True {
                  }
                }
                n161 = call-poly "_DServerSetAttributeValue.vi"("value"=w220, "client request"=w219) -> ()  [unwired: 3 in, 1 out]
              }
              frame "devShortImage" {
                # "return last written value or a random one in \n  case the attribute has never been written"
                n162 = global read "AttributesDataStorage.vi" "i16i"() -> (w232:i16[][])
                n163 = Array Size(array=w232) -> (size(s)=w229:i32[])
                n164 = Index Array(array=w229, index=0) -> (element=w231:i32)
                n165 = Not Equal To 0?(x=w231) -> (x != 0?=w228:bool)
                n166 = case shown="False" w228 {
                  tunnel: [w233 w234] -> w226
                  tunnel: w232 -> [_ w234]
                  frame False {
                    n167 = call-poly "Random2DArray.vi"() -> ("random array"=w233:i16[][])  [unwired: 2 in]
                  }
                  frame True {
                  }
                }
                n168 = call-poly "_DServerSetAttributeValue.vi"("value"=w226, "client request"=w227) -> ()  [unwired: 3 in, 1 out]
              }
              frame "devShortScalar" {
                # "return last written value or a random one in \n  case the attribute has never been written"
                n169 = global read "AttributesDataStorage.vi" "i16"() -> (w237:i16)
                n170 = Not Equal To 0?(x=w237) -> (x != 0?=w238:bool)
                n171 = case shown="False" w238 {
                  tunnel: [w239 w240] -> w236
                  tunnel: w237 -> [_ w240]
                  frame False {
                    n172 = call-poly "RandomScalar.vi"() -> ("random value"=w239:i16)  [unwired: 1 in]
                  }
                  frame True {
                  }
                }
                n173 = call-poly "_DServerSetAttributeValue.vi"("value"=w236, "client request"=w235) -> ()  [unwired: 3 in, 1 out]
              }
              frame "devShortSpectrum" {
                # "return last written value or a random one in \n  case the attribute has never been written"
                n174 = global read "AttributesDataStorage.vi" "i16sp"() -> (w243:i16[])
                n175 = Array Size(array=w243) -> (size(s)=w244:i32)
                n176 = Not Equal To 0?(x=w244) -> (x != 0?=w245:bool)
                n177 = case shown="False" w245 {
                  tunnel: [w246 w247] -> w241
                  tunnel: w243 -> [_ w247]
                  frame False {
                    n178 = call-poly "Random1DArray.vi"() -> ("array"=w246:i16[])  [unwired: 2 in]
                  }
                  frame True {
                  }
                }
                n179 = call-poly "_DServerSetAttributeValue.vi"("value"=w241, "client request"=w242) -> ()  [unwired: 3 in, 1 out]
              }
              frame "devStateImage" {
                n180 = global read "AttributesDataStorage.vi" "state"() -> (w250:T6)
                n181 = Initialize Array(w250, 32 ("dimension size"), 32 ("dimension size")) -> (w249:T6[][])
                n182 = call-poly "_DServerSetAttributeValue.vi"("value"=w249, "client request"=w248) -> ()  [unwired: 3 in, 1 out]
              }
              frame "devStateScalar" {
                n183 = global read "AttributesDataStorage.vi" "state"() -> (w254:T6)
                n184 = call-poly "_DServerSetAttributeValue.vi"("value"=w254, "client request"=w253) -> ()  [unwired: 3 in, 1 out]
              }
              frame "devStateSpectrum" {
                n185 = global read "AttributesDataStorage.vi" "state"() -> (w257:T6)
                n186 = Initialize Array(w257, 32 ("dimension size")) -> (w256:T6[])
                n187 = call-poly "_DServerSetAttributeValue.vi"("value"=w256, "client request"=w255) -> ()  [unwired: 3 in, 1 out]
              }
              frame "devStringImage" {
                # "return last written value or a random one in \n  case the attribute has never been written"
                n188 = global read "AttributesDataStorage.vi" "stri"() -> (w265:string[][])
                n189 = Array Size(array=w265) -> (size(s)=w262:i32[])
                n190 = Index Array(array=w262, index=0) -> (element=w264:i32)
                n191 = Not Equal To 0?(x=w264) -> (x != 0?=w261:bool)
                n192 = case shown="False" w261 {
                  tunnel: [w266 w270] -> w260
                  tunnel: w265 -> [_ w270]
                  frame False {
                    w267 = 32 ("dimension size")
                    n193 = call "RandomValue.vi"() -> ("random value"=w269:dbl)  [unwired: 1 in]
                    n194 = Number To Hexadecimal String(2:w269) -> (0:w268:string)  [unwired: 1 in]
                    n195 = Initialize Array(w268, w267, w267) -> (w266:string[][])
                  }
                  frame True {
                  }
                }
                n196 = call-poly "_DServerSetAttributeValue.vi"("value"=w260, "client request"=w259) -> ()  [unwired: 3 in, 1 out]
              }
              frame "devStringScalar" {
                # "return last written value or a random one in \n  case the attribute has never been written"
                n197 = global read "AttributesDataStorage.vi" "str"() -> (w275:string)
                n198 = String Length(string=w275) -> (length=w273:i32)
                n199 = Not Equal To 0?(x=w273) -> (x != 0?=w274:bool)
                n200 = case shown="False" w274 {
                  tunnel: [w276 w277] -> w272
                  tunnel: w275 -> [_ w277]
                  frame False {
                    n201 = call-poly "RandomScalar.vi"() -> ("random value"=w276:string)  [unwired: 1 in]
                  }
                  frame True {
                  }
                }
                n202 = call-poly "_DServerSetAttributeValue.vi"("value"=w272, "client request"=w271) -> ()  [unwired: 3 in, 1 out]
              }
              frame "devStringSpectrum" {
                # "return last written value or a random one in \n  case the attribute has never been written"
                n203 = global read "AttributesDataStorage.vi" "strsp"() -> (w282:string[])
                n204 = Array Size(array=w282) -> (size(s)=w281:i32)
                n205 = Not Equal To 0?(x=w281) -> (x != 0?=w280:bool)
                n206 = case shown="True" w280 {
                  tunnel: [w283 w287] -> w279
                  tunnel: w282 -> [_ w287]
                  frame False {
                    n207 = call "RandomValue.vi"() -> ("random value"=w285:dbl)  [unwired: 1 in]
                    n208 = Number To Hexadecimal String(2:w285) -> (0:w284:string)  [unwired: 1 in]
                    n209 = Initialize Array(w284, 32 ("dimension size")) -> (w283:string[])
                  }
                  frame True {
                  }
                }
                n210 = call-poly "_DServerSetAttributeValue.vi"("value"=w279, "client request"=w278) -> ()  [unwired: 3 in, 1 out]
              }
              frame "devUCharImage" {
                # "return last written value or a random one in \n  case the attribute has never been written"
                n211 = global read "AttributesDataStorage.vi" "u8i"() -> (w294:u8[][])
                n212 = Array Size(array=w294) -> (size(s)=w291:i32[])
                n213 = Index Array(array=w291, index=0) -> (element=w293:i32)
                n214 = Not Equal To 0?(x=w293) -> (x != 0?=w290:bool)
                n215 = case shown="False" w290 {
                  tunnel: [w295 w296] -> w289
                  tunnel: w294 -> [_ w296]
                  frame False {
                    n216 = call-poly "Random2DArray.vi"() -> ("random array"=w295:u8[][])  [unwired: 2 in]
                  }
                  frame True {
                  }
                }
                n217 = call-poly "_DServerSetAttributeValue.vi"("value"=w289, "client request"=w288) -> ()  [unwired: 3 in, 1 out]
              }
              frame "devUCharScalar" {
                # "return last written value or a random one in \n  case the attribute has never been written"
                n218 = global read "AttributesDataStorage.vi" "u8"() -> (w298:u8)
                n219 = Not Equal To 0?(x=w298) -> (x != 0?=w300:bool)
                n220 = case shown="False" w300 {
                  tunnel: [w301 w302] -> w299
                  tunnel: w298 -> [_ w302]
                  frame False {
                    n221 = call-poly "RandomScalar.vi"() -> ("random value"=w301:u8)  [unwired: 1 in]
                  }
                  frame True {
                  }
                }
                n222 = call-poly "_DServerSetAttributeValue.vi"("value"=w299, "client request"=w297) -> ()  [unwired: 3 in, 1 out]
              }
              frame "devUCharSpectrum" {
                # "return last written value or a random one in \n  case the attribute has never been written"
                n223 = global read "AttributesDataStorage.vi" "u8sp"() -> (w305:u8[])
                n224 = Array Size(array=w305) -> (size(s)=w306:i32)
                n225 = Not Equal To 0?(x=w306) -> (x != 0?=w307:bool)
                n226 = case shown="False" w307 {
                  tunnel: [w308 w309] -> w303
                  tunnel: w305 -> [_ w309]
                  frame False {
                    n227 = call-poly "Random1DArray.vi"() -> ("array"=w308:u8[])  [unwired: 2 in]
                  }
                  frame True {
                  }
                }
                n228 = call-poly "_DServerSetAttributeValue.vi"("value"=w303, "client request"=w304) -> ()  [unwired: 3 in, 1 out]
              }
              frame "devULong64Image" {
                # "return last written value or a random one in \n  case the attribute has never been written"
                n229 = global read "AttributesDataStorage.vi" "u64i"() -> (w316:u64[][])
                n230 = Array Size(array=w316) -> (size(s)=w313:i32[])
                n231 = Index Array(array=w313, index=0) -> (element=w315:i32)
                n232 = Not Equal To 0?(x=w315) -> (x != 0?=w312:bool)
                n233 = case shown="False" w312 {
                  tunnel: [w317 w318] -> w311
                  tunnel: w316 -> [_ w318]
                  frame False {
                    n234 = call-poly "Random2DArray.vi"() -> ("random array"=w317:i64[][])  [unwired: 2 in]
                  }
                  frame True {
                  }
                }
                n235 = call-poly "_DServerSetAttributeValue.vi"("value"=w311, "client request"=w310) -> ()  [unwired: 3 in, 1 out]
              }
              frame "devULong64Scalar" {
                # "return last written value or a random one in \n  case the attribute has never been written"
                n236 = global read "AttributesDataStorage.vi" "u64"() -> (w321:u64)
                n237 = Not Equal To 0?(x=w321) -> (x != 0?=w322:bool)
                n238 = case shown="False" w322 {
                  tunnel: [w323 w324] -> w320
                  tunnel: w321 -> [_ w324]
                  frame False {
                    n239 = call-poly "RandomScalar.vi"() -> ("random value"=w323:u64)  [unwired: 1 in]
                  }
                  frame True {
                  }
                }
                n240 = call-poly "_DServerSetAttributeValue.vi"("value"=w320, "client request"=w319) -> ()  [unwired: 3 in, 1 out]
              }
              frame "devULong64Spectrum" {
                # "return last written value or a random one in \n  case the attribute has never been written"
                n241 = global read "AttributesDataStorage.vi" "u64sp"() -> (w327:u64[])
                n242 = Array Size(array=w327) -> (size(s)=w328:i32)
                n243 = Not Equal To 0?(x=w328) -> (x != 0?=w329:bool)
                n244 = case shown="False" w329 {
                  tunnel: [w330 w331] -> w326
                  tunnel: w327 -> [_ w331]
                  frame False {
                    n245 = call-poly "Random1DArray.vi"() -> ("array"=w330:u64[])  [unwired: 2 in]
                  }
                  frame True {
                  }
                }
                n246 = call-poly "_DServerSetAttributeValue.vi"("value"=w326, "client request"=w325) -> ()  [unwired: 3 in, 1 out]
              }
              frame "devULongImage" {
                # "return last written value or a random one in \n  case the attribute has never been written"
                n247 = global read "AttributesDataStorage.vi" "u32i"() -> (w338:u32[][])
                n248 = Array Size(array=w338) -> (size(s)=w335:i32[])
                n249 = Index Array(array=w335, index=0) -> (element=w337:i32)
                n250 = Not Equal To 0?(x=w337) -> (x != 0?=w334:bool)
                n251 = case shown="False" w334 {
                  tunnel: [w339 w340] -> w333
                  tunnel: w338 -> [_ w340]
                  frame False {
                    n252 = call-poly "Random2DArray.vi"() -> ("random array"=w339:u32[][])  [unwired: 2 in]
                  }
                  frame True {
                  }
                }
                n253 = call-poly "_DServerSetAttributeValue.vi"("value"=w333, "client request"=w332) -> ()  [unwired: 3 in, 1 out]
              }
              frame "devULongScalar" {
                # "return last written value or a random one in \n  case the attribute has never been written"
                n254 = global read "AttributesDataStorage.vi" "u32"() -> (w343:u32)
                n255 = Not Equal To 0?(x=w343) -> (x != 0?=w344:bool)
                n256 = case shown="False" w344 {
                  tunnel: [w345 w346] -> w342
                  tunnel: w343 -> [_ w346]
                  frame False {
                    n257 = call-poly "RandomScalar.vi"() -> ("random value"=w345:u32)  [unwired: 1 in]
                  }
                  frame True {
                  }
                }
                n258 = call-poly "_DServerSetAttributeValue.vi"("value"=w342, "client request"=w341) -> ()  [unwired: 3 in, 1 out]
              }
              frame "devULongSpectrum" {
                # "return last written value or a random one in \n  case the attribute has never been written"
                n259 = global read "AttributesDataStorage.vi" "u32sp"() -> (w349:u32[])
                n260 = Array Size(array=w349) -> (size(s)=w350:i32)
                n261 = Not Equal To 0?(x=w350) -> (x != 0?=w351:bool)
                n262 = case shown="False" w351 {
                  tunnel: [w352 w353] -> w348
                  tunnel: w349 -> [_ w353]
                  frame False {
                    n263 = call-poly "Random1DArray.vi"() -> ("array"=w352:u32[])  [unwired: 2 in]
                  }
                  frame True {
                  }
                }
                n264 = call-poly "_DServerSetAttributeValue.vi"("value"=w348, "client request"=w347) -> ()  [unwired: 3 in, 1 out]
              }
              frame "devUShortImage" {
                # "return last written value or a random one in \n  case the attribute has never been written"
                n265 = global read "AttributesDataStorage.vi" "u16i"() -> (w360:u16[][])
                n266 = Array Size(array=w360) -> (size(s)=w357:i32[])
                n267 = Index Array(array=w357, index=0) -> (element=w359:i32)
                n268 = Not Equal To 0?(x=w359) -> (x != 0?=w356:bool)
                n269 = case shown="False" w356 {
                  tunnel: [w361 w362] -> w355
                  tunnel: w360 -> [_ w362]
                  frame False {
                    n270 = call-poly "Random2DArray.vi"() -> ("random array"=w361:u16[][])  [unwired: 2 in]
                  }
                  frame True {
                  }
                }
                n271 = call-poly "_DServerSetAttributeValue.vi"("value"=w355, "client request"=w354) -> ()  [unwired: 3 in, 1 out]
              }
              frame "devUShortScalar" {
                # "return last written value or a random one in \n  case the attribute has never been written"
                n272 = global read "AttributesDataStorage.vi" "u16"() -> (w365:u16)
                n273 = Not Equal To 0?(x=w365) -> (x != 0?=w366:bool)
                n274 = case shown="False" w366 {
                  tunnel: [w367 w368] -> w364
                  tunnel: w365 -> [_ w368]
                  frame False {
                    n275 = call-poly "RandomScalar.vi"() -> ("random value"=w367:u16)  [unwired: 1 in]
                  }
                  frame True {
                  }
                }
                n276 = call-poly "_DServerSetAttributeValue.vi"("value"=w364, "client request"=w363) -> ()  [unwired: 3 in, 1 out]
              }
              frame "devUShortSpectrum" {
                # "return last written value or a random one in \n  case the attribute has never been written"
                n277 = global read "AttributesDataStorage.vi" "u16sp"() -> (w371:u16[])
                n278 = Array Size(array=w371) -> (size(s)=w372:i32)
                n279 = Not Equal To 0?(x=w372) -> (x != 0?=w373:bool)
                n280 = case shown="False" w373 {
                  tunnel: [w374 w375] -> w370
                  tunnel: w371 -> [_ w375]
                  frame False {
                    n281 = call-poly "Random1DArray.vi"() -> ("array"=w374:u16[])  [unwired: 2 in]
                  }
                  frame True {
                  }
                }
                n282 = call-poly "_DServerSetAttributeValue.vi"("value"=w370, "client request"=w369) -> ()  [unwired: 3 in, 1 out]
              }
              frame "noReplyAttribute" {
                # "we voluntarily don't reply to this request in order to observe the behavior of the Tango binding to such a situation - we expect the waiter (i.e. the thread handling the client request) to timeout and leave the place - the tango device will block (i.e. will not be able to handle another request) until the timeout expires - we consequently understand easily why we should reply to any single request - see _DServerRequestAcknowledgement.vi  -  the _DServerUnimplementedRequest.vi can also be temporary used to deal with \"not yet implemented\" features - see the \"default\" case for an example"
              }
              frame "slowReplyAttribute" {
                # "delay reply to see the timeout mechanism in action"
                n283 = flat-sequence {
                  tunnel: [w378] -> w377
                  tunnel: w376 -> [w378]
                  tunnel: w377 -> [w382]
                  frame #0 {
                    n284 = property on="Device Tmo (in sec)" class="DigNum (strict)"() -> ("Value"=w381:dbl)  [unwired: 2 in, 2 out]
                    n285 = Multiply(x=w381, y=1000.0) -> (x*y=w379:dbl)
                    n286 = Wait (ms)(milliseconds to wait=w379) -> ()  [unwired: 1 out]
                  }
                  frame #1 {
                    n287 = call-poly "Random1DArray.vi"() -> ("array"=w383:i32[])  [unwired: 2 in]
                    n288 = call-poly "_DServerSetAttributeValue.vi"("value"=w383, "client request"=w382) -> ()  [unwired: 3 in, 1 out]
                  }
                }
              }
              frame "State" {
                # "pseudo random state"
                n289 = Tick Count (ms)() -> (millisecond timer value=w386:u32)
                n290 = Quotient & Remainder(x=w386, y=u32 2) -> (x-y*floor(x/y)=w388:u32)  [unwired: 1 out]
                n291 = Equal To 0?(x=w388) -> (x = 0?=w387:bool)
                n292 = case shown="True" w387 {
                  tunnel: [_TangoState_t."OFF" ("Tango Device State") _TangoState_t."ON" ("Tango Device State")] -> w385
                  frame False {
                  }
                  frame True {
                  }
                }
                "State" <- w385
                n293 = call-poly "_DServerSetAttributeValue.vi"("value"=w385, "client request"=w384) -> ()  [unwired: 3 in, 1 out]
              }
              frame "Status" {
                n294 = property on="Tango Device State 1.1" class="Enum (strict)"() -> ("Value"=w394:T6)  [unwired: 2 in, 2 out]
                n295 = call "_TangoStateName.vi"("State"=w394) -> ("State Name"=w393:string)
                n296 = call-poly "_DServerSetAttributeValue.vi"("value"=w393, "client request"=w392) -> ()  [unwired: 3 in, 1 out]
              }
              frame "systematicErrorAttribute" {
                # "the acknowledgement VI can also be used to throw an \nexception that will be caught by the Tango client"
                n297 = call "_DServerRequestAcknowledgement.vi"("error string"="this is a systematic error!", "error code"=-1, "client request"=w397) -> ()  [unwired: 4 in, 1 out]
              }
              frame Default {
                # "oops, this client request is not implemented"
                n298 = call "_DServerUnimplementedRequest.vi"("client request"=w398) -> ()  [unwired: 2 in, 1 out]
              }
            }
          }
          frame "WRITE_ATTR" {
            n299 = case shown="\"devStringScalar\"" w400 {
              tunnel: w399 -> [w401 w404 w407 w410 w413 w416 w419 w422 w425 w428 w431 w434 w437 w440 w443 w446 w449 w452 w455 w458 w461 w464 w467 w471 w473 w476 w479 w482 w485 w488 w491 w494 w497 w500 w503 w506 w509 w512]
              frame "devBooleanImage" {
                n300 = call-poly "_DServerGetAttributeValue.vi"("client request"=w401) -> ("attribute value"=w403:bool[][], "client request"=w402:T1)
                n301 = call "_DServerRequestAcknowledgement.vi"("client request"=w402) -> ()  [unwired: 6 in, 1 out]
                n302 = global write "AttributesDataStorage.vi" "booli"(w403) -> ()
              }
              frame "devBooleanScalar" {
                n303 = call-poly "_DServerGetAttributeValue.vi"("client request"=w404) -> ("attribute value"=w406:bool, "client request"=w405:T1)
                n304 = call "_DServerRequestAcknowledgement.vi"("client request"=w405) -> ()  [unwired: 6 in, 1 out]
                n305 = global write "AttributesDataStorage.vi" "bool"(w406) -> ()
              }
              frame "devBooleanSpectrum" {
                n306 = call-poly "_DServerGetAttributeValue.vi"("client request"=w407) -> ("attribute value"=w409:bool[], "client request"=w408:T1)
                n307 = call "_DServerRequestAcknowledgement.vi"("client request"=w408) -> ()  [unwired: 6 in, 1 out]
                n308 = global write "AttributesDataStorage.vi" "boolsp"(w409) -> ()
              }
              frame "devDoubleImage" {
                n309 = call-poly "_DServerGetAttributeValue.vi"("client request"=w410) -> ("attribute value"=w412:dbl[][], "client request"=w411:T1)
                n310 = call "_DServerRequestAcknowledgement.vi"("client request"=w411) -> ()  [unwired: 6 in, 1 out]
                n311 = global write "AttributesDataStorage.vi" "dbli"(w412) -> ()
              }
              frame "devDoubleScalar" {
                n312 = call-poly "_DServerGetAttributeValue.vi"("client request"=w413) -> ("attribute value"=w415:dbl, "client request"=w414:T1)
                n313 = call "_DServerRequestAcknowledgement.vi"("client request"=w414) -> ()  [unwired: 6 in, 1 out]
                n314 = global write "AttributesDataStorage.vi" "dbl"(w415) -> ()
                n315 = property on="devDoubleScalar" class="Knob (strict)"("Val(Sgnl)"=w415) -> ()  [unwired: 2 in, 2 out]
              }
              frame "devDoubleSpectrum" {
                n316 = call-poly "_DServerGetAttributeValue.vi"("client request"=w416) -> ("attribute value"=w418:dbl[], "client request"=w417:T1)
                n317 = call "_DServerRequestAcknowledgement.vi"("client request"=w417) -> ()  [unwired: 6 in, 1 out]
                n318 = global write "AttributesDataStorage.vi" "dblsp"(w418) -> ()
              }
              frame "devFloatImage" {
                n319 = call-poly "_DServerGetAttributeValue.vi"("client request"=w419) -> ("attribute value"=w421:sgl[][], "client request"=w420:T1)
                n320 = call "_DServerRequestAcknowledgement.vi"("client request"=w420) -> ()  [unwired: 6 in, 1 out]
                n321 = global write "AttributesDataStorage.vi" "sgli"(w421) -> ()
              }
              frame "devFloatScalar" {
                n322 = call-poly "_DServerGetAttributeValue.vi"("client request"=w422) -> ("attribute value"=w424:sgl, "client request"=w423:T1)
                n323 = call "_DServerRequestAcknowledgement.vi"("client request"=w423) -> ()  [unwired: 6 in, 1 out]
                n324 = global write "AttributesDataStorage.vi" "sgl"(w424) -> ()
              }
              frame "devFloatSpectrum" {
                n325 = call-poly "_DServerGetAttributeValue.vi"("client request"=w425) -> ("attribute value"=w427:sgl[], "client request"=w426:T1)
                n326 = call "_DServerRequestAcknowledgement.vi"("client request"=w426) -> ()  [unwired: 6 in, 1 out]
                n327 = global write "AttributesDataStorage.vi" "sglsp"(w427) -> ()
              }
              frame "devLong64Image" {
                n328 = call-poly "_DServerGetAttributeValue.vi"("client request"=w428) -> ("attribute value"=w430:i64[][], "client request"=w429:T1)
                n329 = call "_DServerRequestAcknowledgement.vi"("client request"=w429) -> ()  [unwired: 6 in, 1 out]
                n330 = global write "AttributesDataStorage.vi" "i64i"(w430) -> ()
              }
              frame "devLong64Scalar" {
                n331 = call-poly "_DServerGetAttributeValue.vi"("client request"=w431) -> ("attribute value"=w433:i64, "client request"=w432:T1)
                n332 = call "_DServerRequestAcknowledgement.vi"("client request"=w432) -> ()  [unwired: 6 in, 1 out]
                n333 = global write "AttributesDataStorage.vi" "i64"(w433) -> ()
              }
              frame "devLong64Spectrum" {
                n334 = call-poly "_DServerGetAttributeValue.vi"("client request"=w434) -> ("attribute value"=w436:i64[], "client request"=w435:T1)
                n335 = call "_DServerRequestAcknowledgement.vi"("client request"=w435) -> ()  [unwired: 6 in, 1 out]
                n336 = global write "AttributesDataStorage.vi" "i64sp"(w436) -> ()
              }
              frame "devLongImage" {
                n337 = call-poly "_DServerGetAttributeValue.vi"("client request"=w437) -> ("attribute value"=w439:i32[][], "client request"=w438:T1)
                n338 = call "_DServerRequestAcknowledgement.vi"("client request"=w438) -> ()  [unwired: 6 in, 1 out]
                n339 = global write "AttributesDataStorage.vi" "i32i"(w439) -> ()
              }
              frame "devLongScalar" {
                n340 = call-poly "_DServerGetAttributeValue.vi"("client request"=w440) -> ("attribute value"=w442:i32, "client request"=w441:T1)
                n341 = call "_DServerRequestAcknowledgement.vi"("client request"=w441) -> ()  [unwired: 6 in, 1 out]
                n342 = global write "AttributesDataStorage.vi" "i32"(w442) -> ()
              }
              frame "devLongSpectrum" {
                n343 = call-poly "_DServerGetAttributeValue.vi"("client request"=w443) -> ("attribute value"=w445:i32[], "client request"=w444:T1)
                n344 = call "_DServerRequestAcknowledgement.vi"("client request"=w444) -> ()  [unwired: 6 in, 1 out]
                n345 = global write "AttributesDataStorage.vi" "i32sp"(w445) -> ()
              }
              frame "devShortImage" {
                n346 = call-poly "_DServerGetAttributeValue.vi"("client request"=w446) -> ("attribute value"=w448:i16[][], "client request"=w447:T1)
                n347 = call "_DServerRequestAcknowledgement.vi"("client request"=w447) -> ()  [unwired: 6 in, 1 out]
                n348 = global write "AttributesDataStorage.vi" "i16i"(w448) -> ()
              }
              frame "devShortScalar" {
                n349 = call-poly "_DServerGetAttributeValue.vi"("client request"=w449) -> ("attribute value"=w451:i16, "client request"=w450:T1)
                n350 = call "_DServerRequestAcknowledgement.vi"("client request"=w450) -> ()  [unwired: 6 in, 1 out]
                n351 = global write "AttributesDataStorage.vi" "i16"(w451) -> ()
              }
              frame "devEnumScalar" {
                n352 = call-poly "_DServerGetAttributeValue.vi"("client request"=w452) -> ("attribute value"=w454:i16, "client request"=w453:T1)
                n353 = global write "AttributesDataStorage.vi" "enum"(w454) -> ()
                n354 = call "_DServerRequestAcknowledgement.vi"("client request"=w453) -> ()  [unwired: 6 in, 1 out]
              }
              frame "devShortSpectrum" {
                n355 = call-poly "_DServerGetAttributeValue.vi"("client request"=w455) -> ("attribute value"=w457:i16[], "client request"=w456:T1)
                n356 = call "_DServerRequestAcknowledgement.vi"("client request"=w456) -> ()  [unwired: 6 in, 1 out]
                n357 = global write "AttributesDataStorage.vi" "i16sp"(w457) -> ()
              }
              frame "devStateImage" {
                n358 = call-poly "_DServerGetAttributeValue.vi"("client request"=w458) -> ("attribute value"=w460:T6[][], "client request"=w459:T1)
                n359 = call "_DServerRequestAcknowledgement.vi"("client request"=w459) -> ()  [unwired: 6 in, 1 out]
                n360 = global write "AttributesDataStorage.vi" "statei"(w460) -> ()
              }
              frame "devStateScalar" {
                n361 = call-poly "_DServerGetAttributeValue.vi"("client request"=w461) -> ("attribute value"=w463:T6, "client request"=w462:T1)
                n362 = call "_DServerRequestAcknowledgement.vi"("client request"=w462) -> ()  [unwired: 6 in, 1 out]
                n363 = global write "AttributesDataStorage.vi" "state"(w463) -> ()
              }
              frame "devStateSpectrum" {
                n364 = call-poly "_DServerGetAttributeValue.vi"("client request"=w464) -> ("attribute value"=w466:T6[], "client request"=w465:T1)
                n365 = call "_DServerRequestAcknowledgement.vi"("client request"=w465) -> ()  [unwired: 6 in, 1 out]
                n366 = global write "AttributesDataStorage.vi" "statesp"(w466) -> ()
              }
              frame "devStringImage" {
                n367 = call-poly "_DServerGetAttributeValue.vi"("client request"=w467) -> ("attribute value"=w469:string[][], "client request"=w468:T1)
                n368 = global write "AttributesDataStorage.vi" "stri"(w469) -> ()
                n369 = call "_DServerRequestAcknowledgement.vi"("client request"=w468) -> ()  [unwired: 6 in, 1 out]
              }
              frame "devStringScalar" {
                n370 = call-poly "_DServerGetAttributeValue.vi"("client request"=w471) -> ("attribute value"=w470:string, "client request"=w472:T1)
                n371 = call "_DServerRequestAcknowledgement.vi"("client request"=w472) -> ()  [unwired: 6 in, 1 out]
                n372 = global write "AttributesDataStorage.vi" "str"(w470) -> ()
              }
              frame "devStringSpectrum" {
                n373 = call-poly "_DServerGetAttributeValue.vi"("client request"=w473) -> ("attribute value"=w475:string[], "client request"=w474:T1)
                n374 = call "_DServerRequestAcknowledgement.vi"("client request"=w474) -> ()  [unwired: 6 in, 1 out]
                n375 = global write "AttributesDataStorage.vi" "strsp"(w475) -> ()
              }
              frame "devUCharImage" {
                n376 = call-poly "_DServerGetAttributeValue.vi"("client request"=w476) -> ("attribute value"=w478:u8[][], "client request"=w477:T1)
                n377 = call "_DServerRequestAcknowledgement.vi"("client request"=w477) -> ()  [unwired: 6 in, 1 out]
                n378 = global write "AttributesDataStorage.vi" "u8i"(w478) -> ()
              }
              frame "devUCharScalar" {
                n379 = call-poly "_DServerGetAttributeValue.vi"("client request"=w479) -> ("attribute value"=w481:u8, "client request"=w480:T1)
                n380 = call "_DServerRequestAcknowledgement.vi"("client request"=w480) -> ()  [unwired: 6 in, 1 out]
                n381 = global write "AttributesDataStorage.vi" "u8"(w481) -> ()
              }
              frame "devUCharSpectrum" {
                n382 = call-poly "_DServerGetAttributeValue.vi"("client request"=w482) -> ("attribute value"=w484:u8[], "client request"=w483:T1)
                n383 = call "_DServerRequestAcknowledgement.vi"("client request"=w483) -> ()  [unwired: 6 in, 1 out]
                n384 = global write "AttributesDataStorage.vi" "u8sp"(w484) -> ()
              }
              frame "devULong64Image" {
                n385 = call-poly "_DServerGetAttributeValue.vi"("client request"=w485) -> ("attribute value"=w487:u64[], "client request"=w486:T1)
                n386 = call "_DServerRequestAcknowledgement.vi"("client request"=w486) -> ()  [unwired: 6 in, 1 out]
                n387 = global write "AttributesDataStorage.vi" "u64sp"(w487) -> ()
              }
              frame "devULong64Scalar" {
                n388 = call-poly "_DServerGetAttributeValue.vi"("client request"=w488) -> ("attribute value"=w490:u64, "client request"=w489:T1)
                n389 = call "_DServerRequestAcknowledgement.vi"("client request"=w489) -> ()  [unwired: 6 in, 1 out]
                n390 = global write "AttributesDataStorage.vi" "u64"(w490) -> ()
              }
              frame "devULong64Spectrum" {
                n391 = call-poly "_DServerGetAttributeValue.vi"("client request"=w491) -> ("attribute value"=w493:u64[], "client request"=w492:T1)
                n392 = call "_DServerRequestAcknowledgement.vi"("client request"=w492) -> ()  [unwired: 6 in, 1 out]
                n393 = global write "AttributesDataStorage.vi" "u64sp"(w493) -> ()
              }
              frame "devULongImage" {
                n394 = call-poly "_DServerGetAttributeValue.vi"("client request"=w494) -> ("attribute value"=w496:u32[][], "client request"=w495:T1)
                n395 = call "_DServerRequestAcknowledgement.vi"("client request"=w495) -> ()  [unwired: 6 in, 1 out]
                n396 = global write "AttributesDataStorage.vi" "u32i"(w496) -> ()
              }
              frame "devULongScalar" {
                n397 = call-poly "_DServerGetAttributeValue.vi"("client request"=w497) -> ("attribute value"=w499:u32, "client request"=w498:T1)
                n398 = call "_DServerRequestAcknowledgement.vi"("client request"=w498) -> ()  [unwired: 6 in, 1 out]
                n399 = global write "AttributesDataStorage.vi" "u32"(w499) -> ()
              }
              frame "devULongSpectrum" {
                n400 = call-poly "_DServerGetAttributeValue.vi"("client request"=w500) -> ("attribute value"=w502:u32[], "client request"=w501:T1)
                n401 = call "_DServerRequestAcknowledgement.vi"("client request"=w501) -> ()  [unwired: 6 in, 1 out]
                n402 = global write "AttributesDataStorage.vi" "u32sp"(w502) -> ()
              }
              frame "devUShortImage" {
                n403 = call-poly "_DServerGetAttributeValue.vi"("client request"=w503) -> ("attribute value"=w505:u16[][], "client request"=w504:T1)
                n404 = call "_DServerRequestAcknowledgement.vi"("client request"=w504) -> ()  [unwired: 6 in, 1 out]
                n405 = global write "AttributesDataStorage.vi" "u16i"(w505) -> ()
              }
              frame "devUShortScalar" {
                n406 = call-poly "_DServerGetAttributeValue.vi"("client request"=w506) -> ("attribute value"=w508:u16, "client request"=w507:T1)
                n407 = call "_DServerRequestAcknowledgement.vi"("client request"=w507) -> ()  [unwired: 6 in, 1 out]
                n408 = global write "AttributesDataStorage.vi" "u16"(w508) -> ()
              }
              frame "devUShortSpectrum" {
                n409 = call-poly "_DServerGetAttributeValue.vi"("client request"=w509) -> ("attribute value"=w511:u16[], "client request"=w510:T1)
                n410 = call "_DServerRequestAcknowledgement.vi"("client request"=w510) -> ()  [unwired: 6 in, 1 out]
                n411 = global write "AttributesDataStorage.vi" "u16sp"(w511) -> ()
              }
              frame Default {
                # "oops, this client request is not implemented"
                n412 = call "_DServerUnimplementedRequest.vi"("client request"=w512) -> ()  [unwired: 2 in, 1 out]
              }
            }
          }
          frame "UNKNOWN_REQUEST", Default {
            n413 = call "_DServerUnimplementedRequest.vi"("client request"=w513) -> ()  [unwired: 2 in, 1 out]
          }
        }
        "Client Request" <- w15
      }
      frame True {
      }
    }
  }
  n414 = call "_DServerStop.vi"("error in"=w2, "dserver evt."=w1) -> ()  [unwired: 1 in, 1 out]
